vi "get_tiff_pixels_size.vi"(8 "error in (no error)":errorcluster, 10 "path_filename in":string, 11 "ScanModeTS090821Circular2D in":refnum<class "ScanModeTS090821Circular2D.lvclass">=refnum) -> (0 "error out":errorcluster, 1 "y_size":dbl, 2 "x_size":dbl, 3 "ScanModeTS090821Circular2D out":refnum<class "ScanModeTS090821Circular2D.lvclass">)   [LabVIEW 2010]
uses:
  main/dlls/saveTiffStack_v02b/ome_dll.dll
  ScanModeTS090821Circular2D.lvclass
panel:
  out "path_filename":string
  out "Output Value":i32
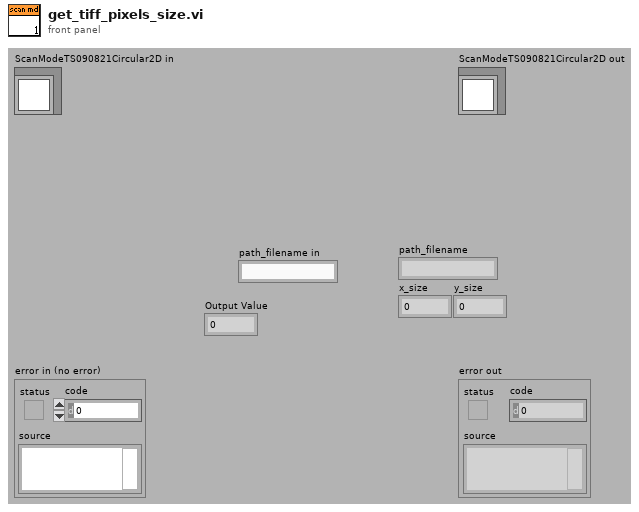
[diagram p1: front panel]
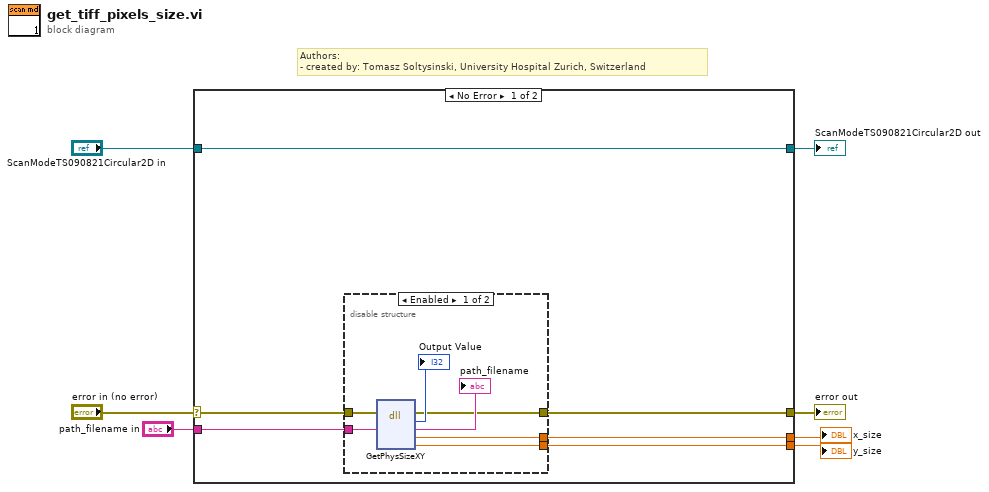
[diagram p0: block diagram]
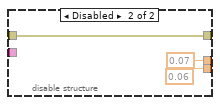
[diagram p2: hidden frame]
diagram:
  # "Authors: \n- created by: Tomasz Soltysinski, University Hospital Zurich, Switzerland"
  n1 = case shown="No Error" "error in (no error)" {
    selector: "error in (no error)" -> [w9 w25]
    tunnel: [w8 w25] -> w6
    tunnel: [w13 w24] -> w4
    tunnel: "ScanModeTS090821Circular2D in" -> [w13 w24]
    tunnel: "path_filename in" -> [w12 _]
    tunnel: [w11 _] -> w2
    tunnel: [w10 _] -> w1
    frame No Error {
      n2 = disable-structure shown="Enabled" {
        disable-tunnel: w12 -> [w20 _]
        disable-tunnel: [w19 0.07 ("x_size")] -> w11
        disable-tunnel: [w18 0.06 ("y_size")] -> w10
        disable-tunnel: w9 -> [w15 w23]
        disable-tunnel: [w14 w23] -> w8
        frame Enabled {
          n3 = dll-call lib="C:/helioscan/main/dlls/saveTiffStack_v02b/ome_dll.dll" fn="GetPhysSizeXY"(error in=w15, "path_filename"=w20) -> (error out=w14:errorcluster, "return type"=→"Output Value":i32, "path_filename"=→"path_filename":string, "x_size"=w19:dbl, "y_size"=w18:dbl)  [unwired: 4 in, 1 out]
        }
        frame Disabled {
        }
      }
    }
    frame Error {
    }
  }
  "error out" <- w6
  "ScanModeTS090821Circular2D out" <- w4
  "x_size" <- w2
  "y_size" <- w1
